vi "graba-eeprom.vi"(0 "Equipo Nº":u8, 1 "Eeprom":string, 2 "COM DATA":T1) -> (6 "error out":errorcluster)   [LabVIEW 2010]
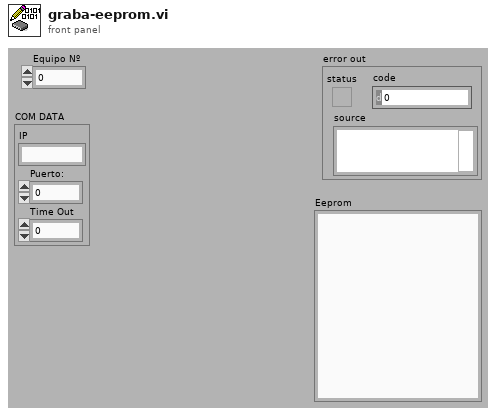
[diagram p1: front panel]
types:
  T1 = cluster{"IP ":string, "Puerto:":u16, "Time Out":u16}
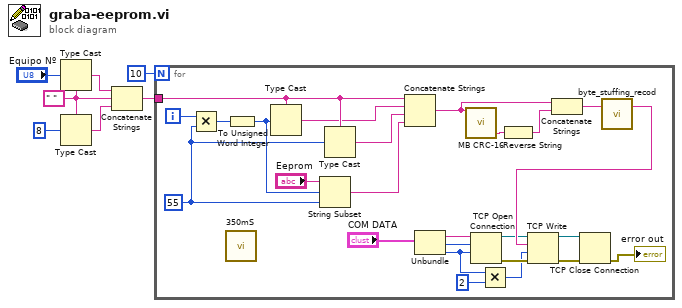
[diagram p0: block diagram]
diagram:
  w2 = " " ("Lectura 2")
  n1 = Type Cast(type=w2, x="Equipo Nº") -> (*(type *) &x=w6:string)
  n2 = Type Cast(type=w2, x=u8 8 ("Comando:")) -> (*(type *) &x=w4:string)
  n3 = Concatenate Strings(w6, w2, w4) -> (w3:string)
  n4 = for {
    N: 10 -> [_]
    tunnel: w3 -> [w28]
    i -> [w29]
    w22 = u16 55 ("BYTES")
    n5 = Multiply(x=w29, y=w22) -> (x*y=w25:i32)
    n6 = call "350mS"() -> ()  [unwired: 11 in, 1 out]
    n7 = To Unsigned Word Integer(number=w25) -> (unsigned 16bit integer=w24:u16)
    n8 = Type Cast(type=w28, x=w24) -> (*(type *) &x=w26:string)
    n9 = String Subset(string="Eeprom", offset (0)=w24, length (rest)=w22) -> (substring=w21:string)
    n10 = Type Cast(type=w28, x=w22) -> (*(type *) &x=w27:string)
    n11 = Concatenate Strings(w28, w26, w27, w21) -> (w23:string)
    n12 = Unbundle("COM DATA") -> ("IP"=w17:string, "Puerto:"=w16:u16, "Time Out"=w11:u16)
    n13 = call "MB CRC-16.vi"("String"=w23) -> ("CRC-16"=w31:string)  [unwired: 2 in, 2 out]
    n14 = TCP Open Connection(address=w17, remote port or service name=w16, timeout ms (60000)=w11) -> (connection ID=w15:refnum<k5>, error out=w14:errorcluster)  [unwired: 2 in]
    n15 = Multiply(x=w11, y=2) -> (x*y=w12:i32)
    n16 = Reverse String(1:w31) -> (0:w32:string)
    n17 = Concatenate Strings(w23, w32) -> (w20:string)
    n18 = call "byte_stuffing_recod.vi"("String IN"=w20) -> ("String OUT"=w19:string)  [unwired: 2 out]
    n19 = TCP Write(connection ID=w15, data in=w19, error in (no error)=w14, 9:w12) -> (connection ID out=w9:refnum<k5>, error out=w8:errorcluster)  [unwired: 1 out]
    n20 = TCP Close Connection(connection ID=w9, error in (no error)=w8) -> (error out=→"error out":errorcluster)  [unwired: 1 in, 1 out]
  }
